vi "bazar.vi"() -> ()   [LabVIEW 2014]
uses:
  <userlib>/AndorSDK3/Data/GetPixelData16.vi
panel:
  out "Photoluminescence versus time":cluster{"X":dbl, "Y":dbl}[](graph)
  in  "Apply Settings":bool
  in  "Centre AOI":bool
  in  "AOI Width":i64
  in  "AOI Height":i64
  in  "Run":bool
  out "Ready":bool
  out "Intensity Graph":u16[][](graph)
  in  "error":errorcluster
  out "AOIStride":i64
  out "Pixel Encoding":string
  in  "PreAmp Gain Control":string(combo)
  out "PixelData":u16[](array[numeric])
  out "ByteData":u8[](array[numeric])
  in  "ExposureTime":dbl=0.1
  out "ImageSizeBytes":i64
  out "Handle":i32
  in  "Set CW Light":bool
  in  "Technical parameters":enum32{"Aardvark", "762 Address", "Errors"}(tab)
  out "Bit Rate":i16
  out "Aardvark Power Enable":bool
  out "Pullup?":bool
  in  "Num Bytes to Fetch (64)":u8=64 min=1
  in  "Address (0x50)":u16=80 max=1023 format="%.0x"
  in  "error in (no error)":errorcluster
  out "error out":errorcluster
  in  "Disabel Output":bool
  out "Light ON":bool
  in  "Enable Ouput":bool
  in  "Dark Time":dbl
  in  "Pulse Period":dbl
  in  "Pulse Width":dbl
  in  "Laser Current (A)":dbl
  in  "Set Config.":bool
  in  "Read Current Config.":bool
  out "Dark Time":dbl
  out "Pulse Period":dbl
  out "Pulse Width":dbl
  out "Laser Current (A)":dbl
  # "Pulsed Light"
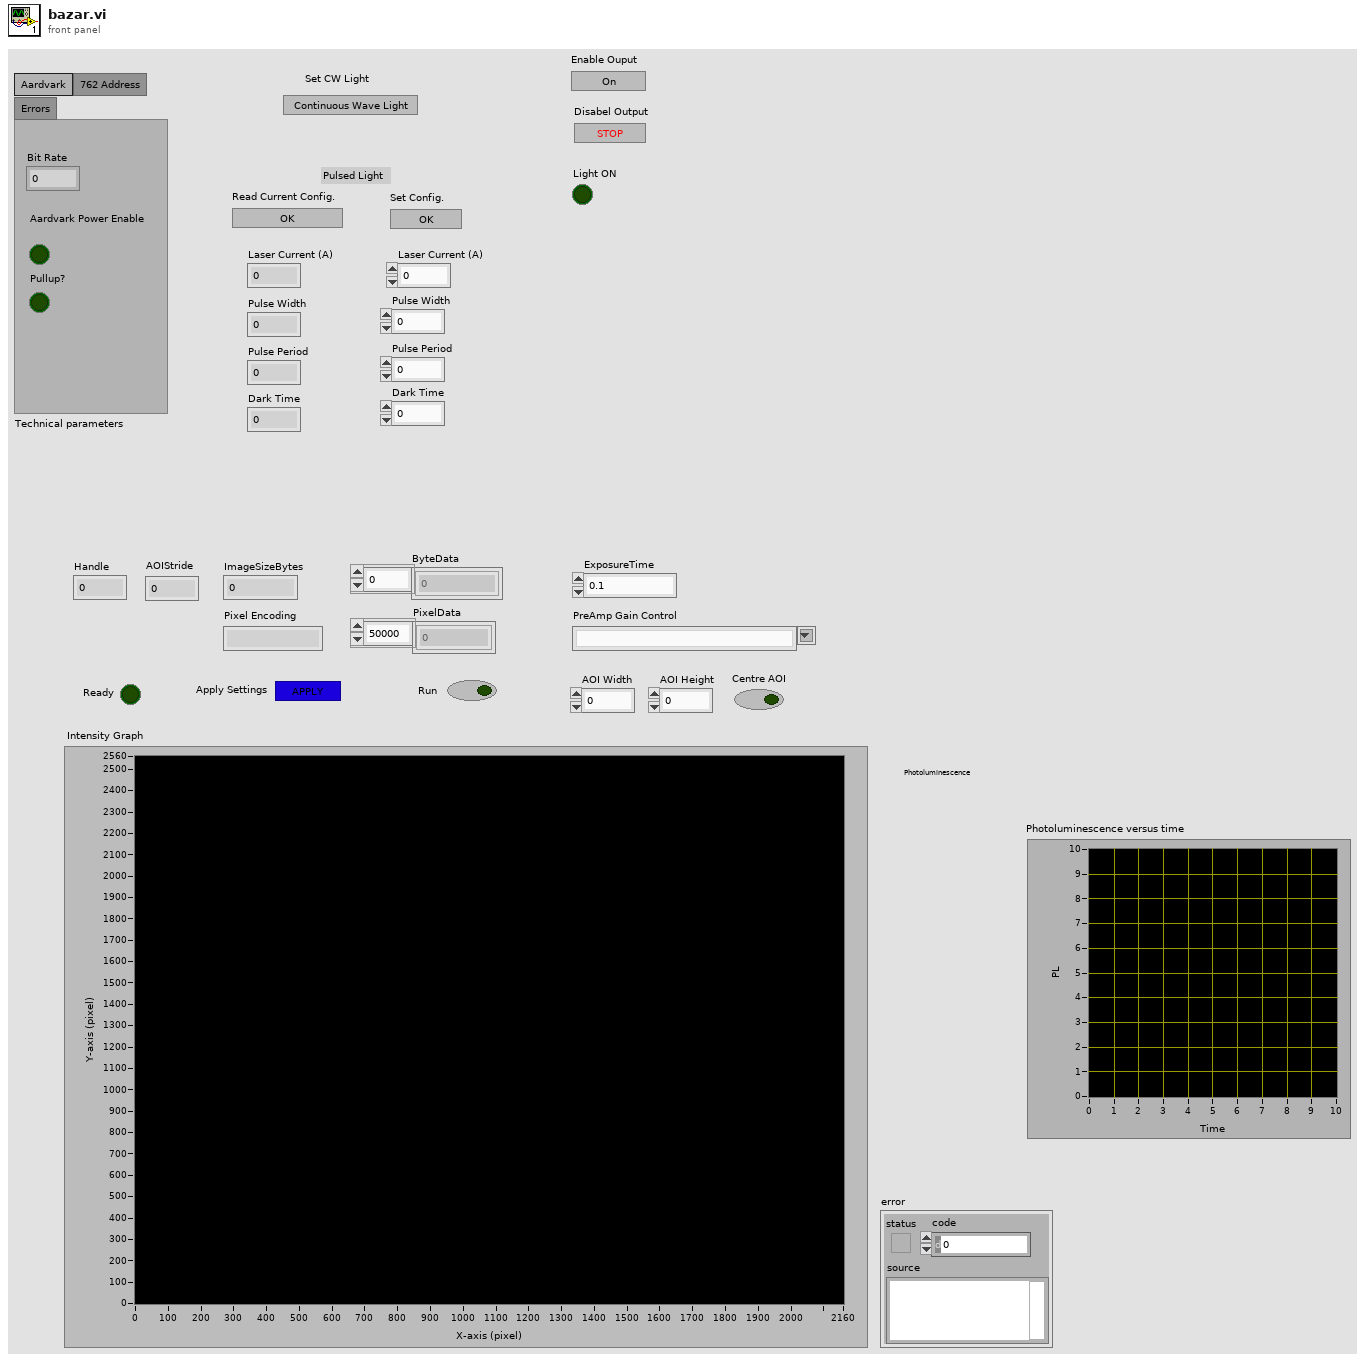
[diagram p1: front panel]
types:
  T1 = enum8{"Enabled", "Disabled", "Disabled and Grayed Out"}
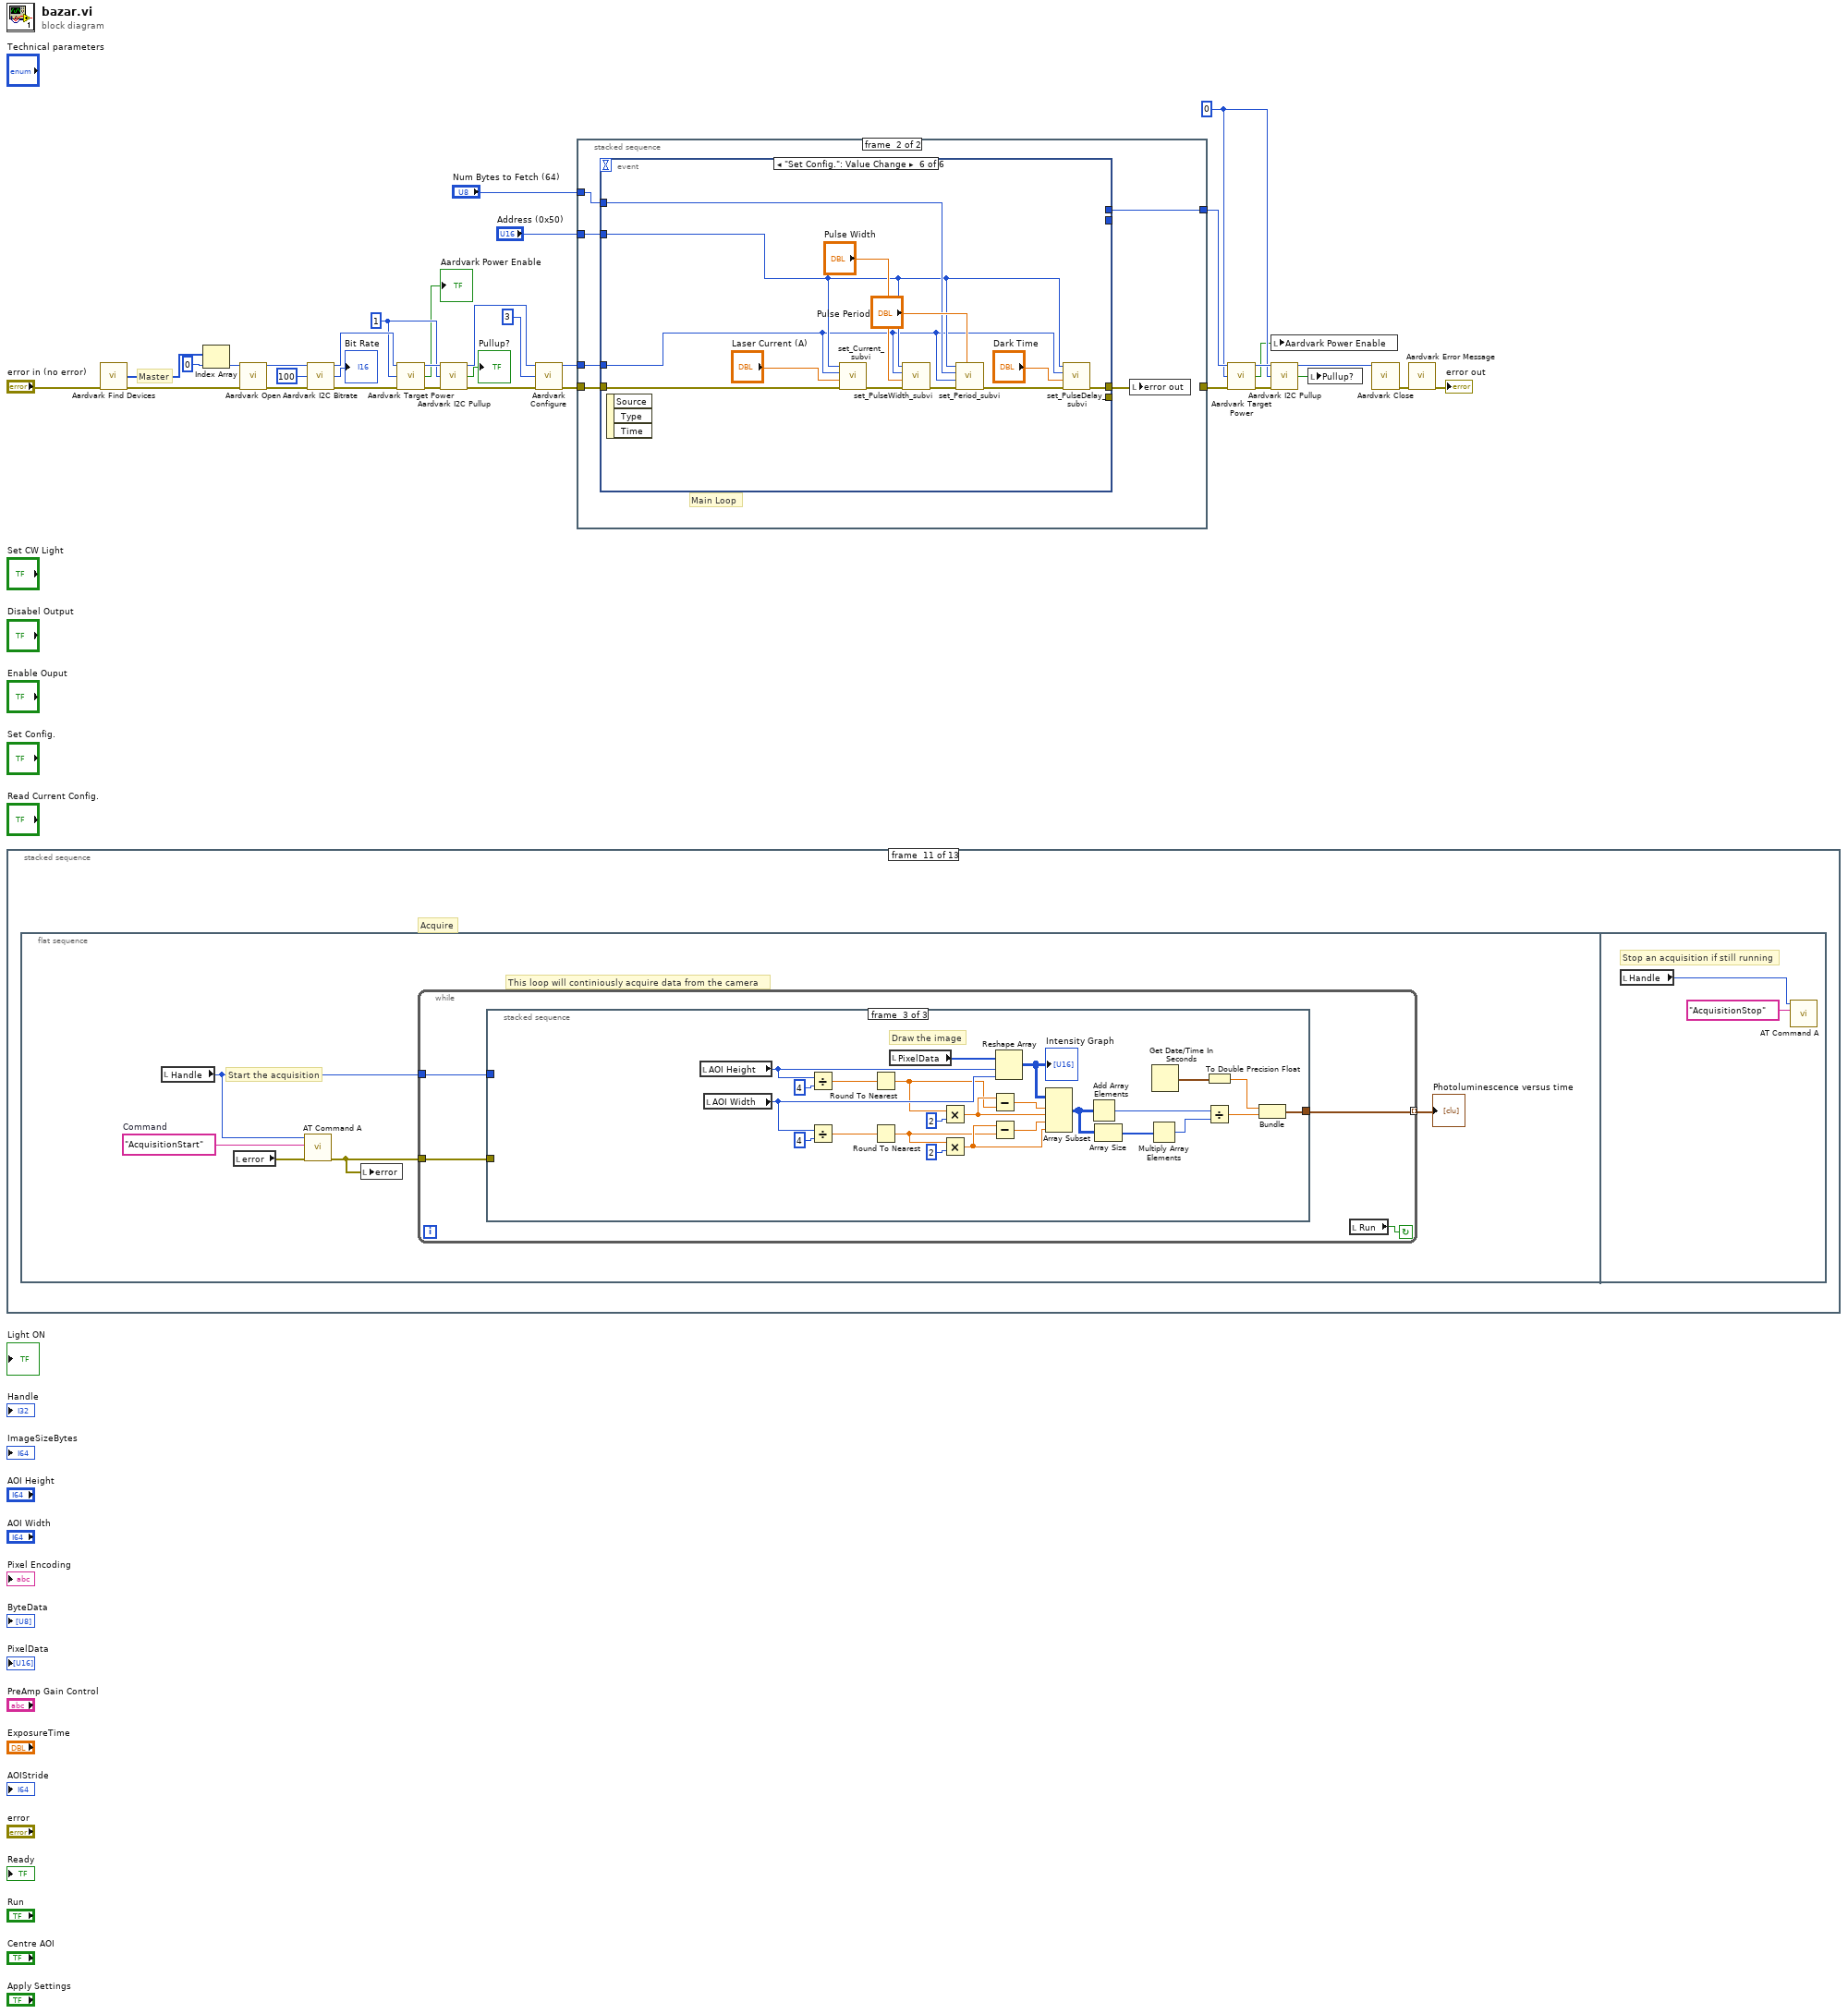
[diagram p0: block diagram]
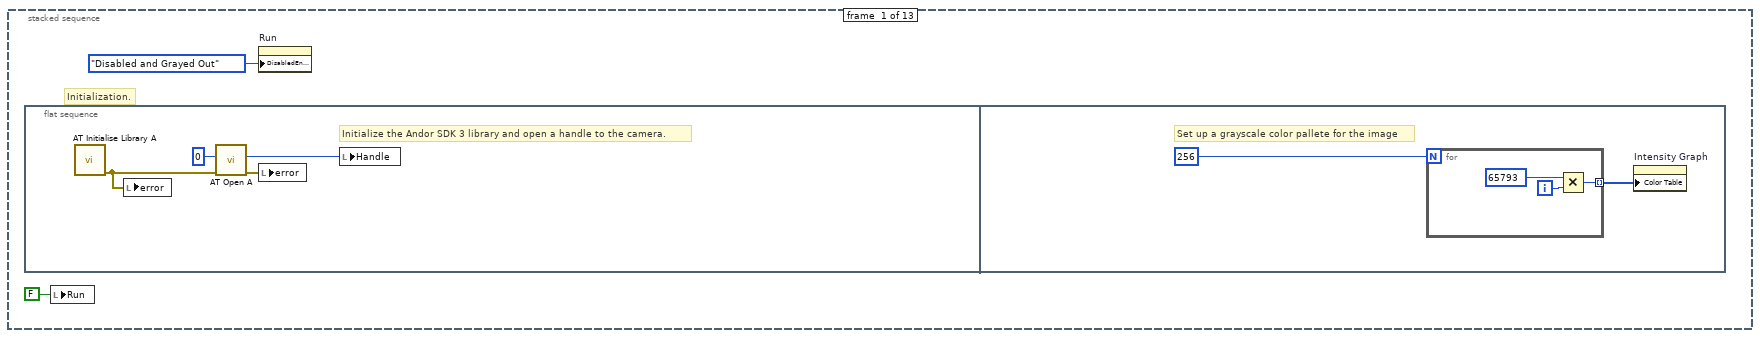
[diagram p2: hidden frame]
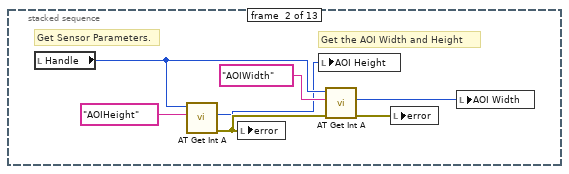
[diagram p3: hidden frame]
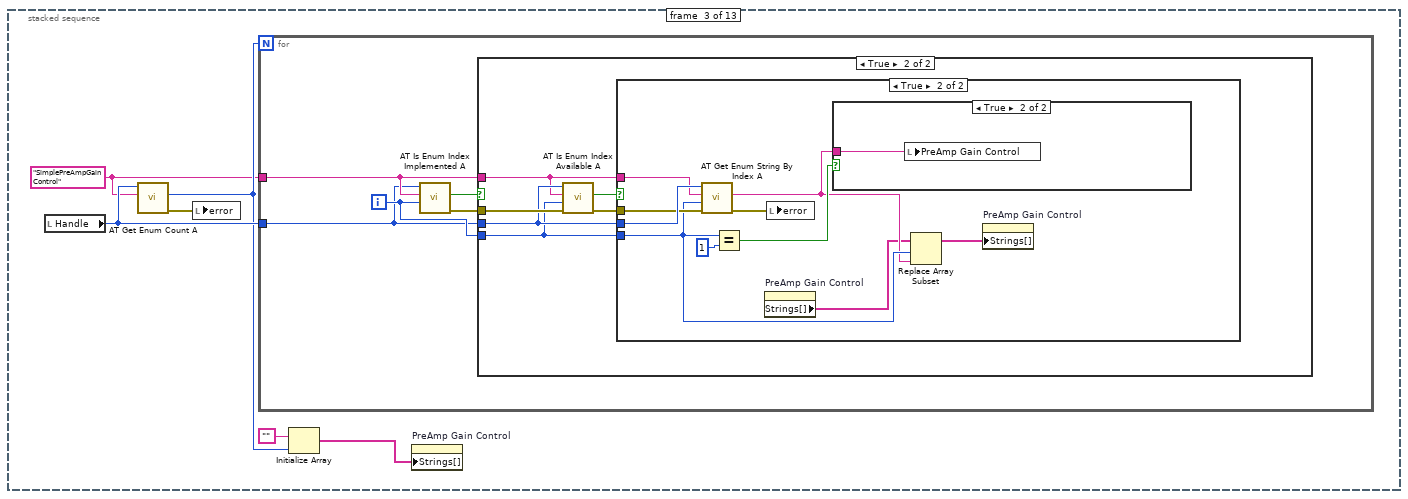
[diagram p4: hidden frame]
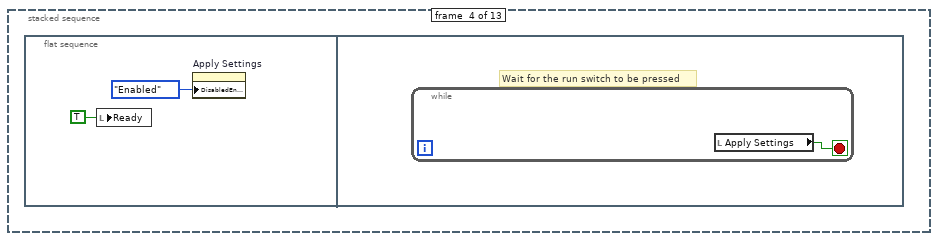
[diagram p8: hidden frame]
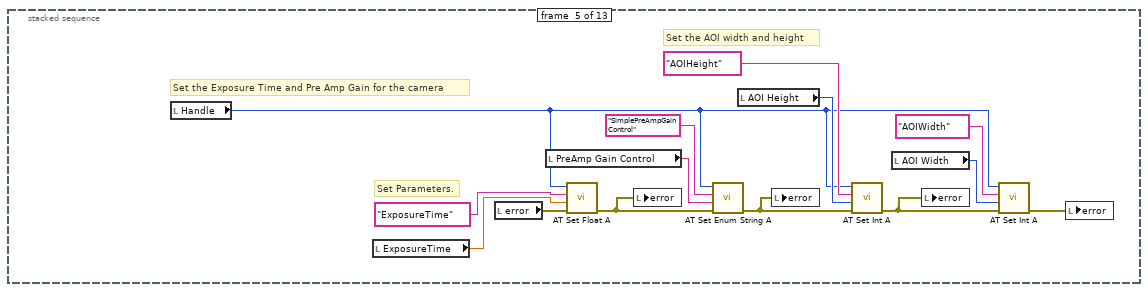
[diagram p9: hidden frame]
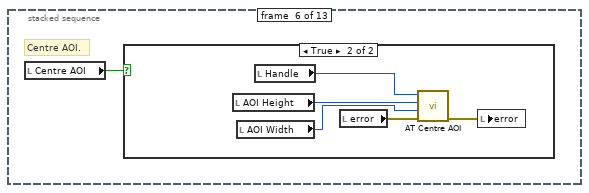
[diagram p10: hidden frame]
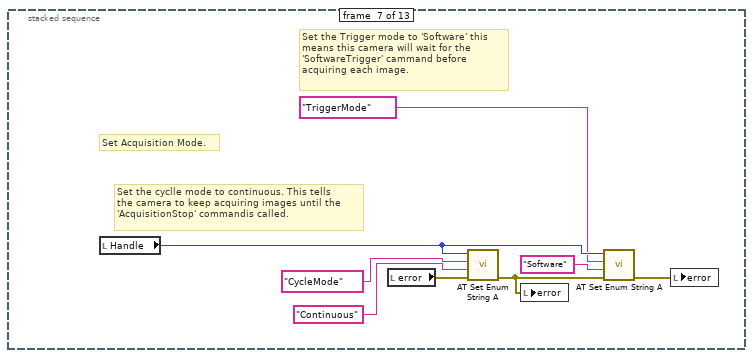
[diagram p12: hidden frame]
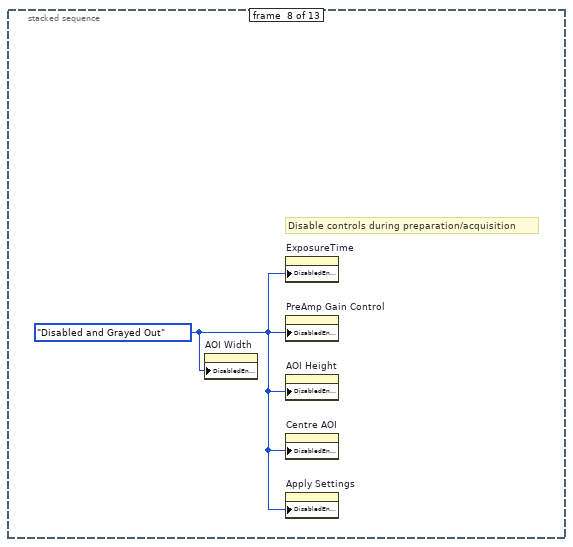
[diagram p13: hidden frame]
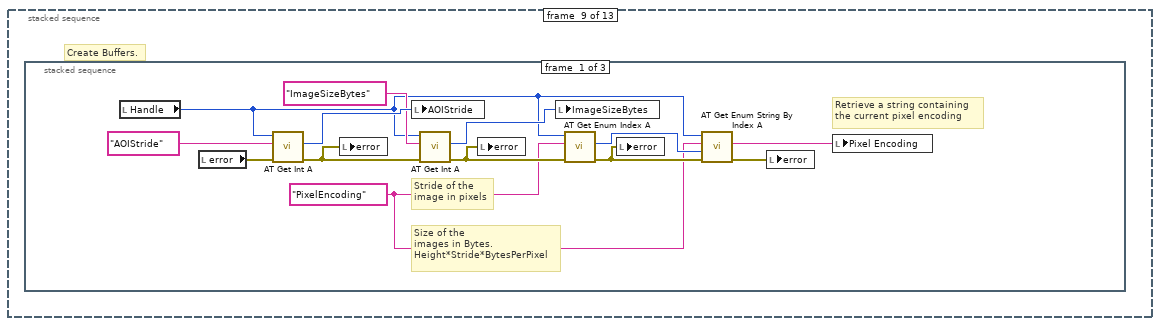
[diagram p14: hidden frame]
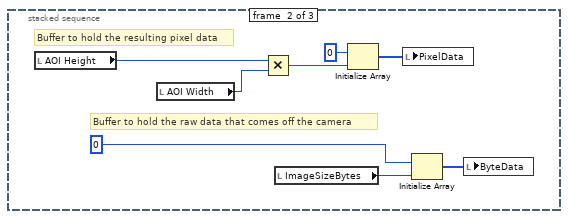
[diagram p15: hidden frame]
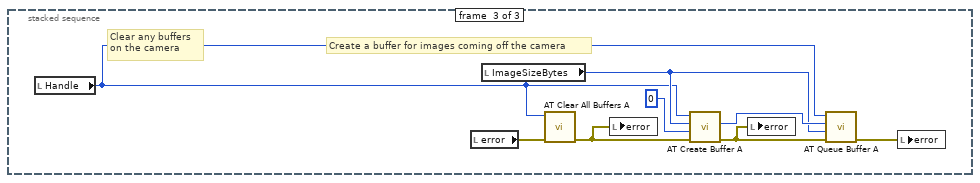
[diagram p16: hidden frame]
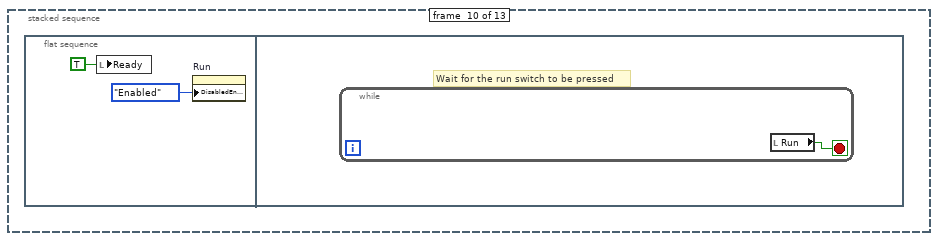
[diagram p17: hidden frame]
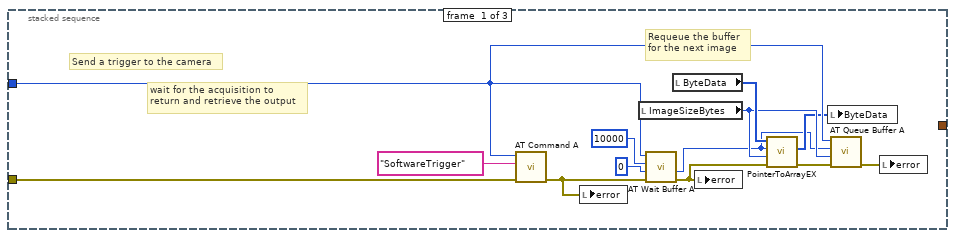
[diagram p18: hidden frame]
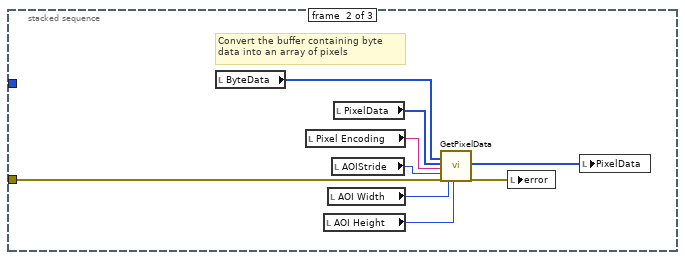
[diagram p19: hidden frame]
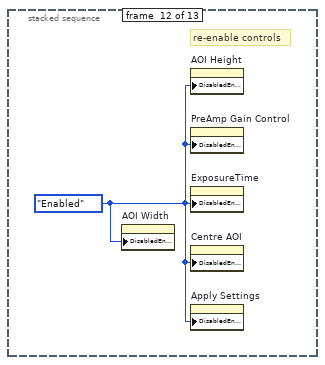
[diagram p20: hidden frame]
diagram:
  w3 = 0
  w13 = 1
  # "Master"
  n1 = stacked-sequence {
    frame #0 {
      # "Initialization."
      n2 = flat-sequence {
        frame #0 {
          # "Initialize the Andor SDK 3 library and open a handle to the camera."
          n3 = call <userlib>:"AT Initialise Library A.vi"() -> ("error out"=w37:errorcluster)  [unwired: 10 in, 1 out]
          n4 = local write "error"(w37) -> ()
          n5 = call <userlib>:"AT Open A.vi"("error in (no error)"=w37, "CameraIndex"=0) -> ("error out"=w36:errorcluster, "Handle"=w38:i32)  [unwired: 7 in, 1 out]
          n6 = local write "error"(w36) -> ()
          n7 = local write "Handle"(w38) -> ()
        }
        frame #1 {
          # "Set up a grayscale color pallete for the image"
          n8 = for {
            N: 256 -> [_]
            tunnel: [w43] -> w40 mode=indexing
            i -> [w44]
            n9 = Multiply(x=65793, y=w44) -> (x*y=w43:i32)
          }
          n10 = property on="Intensity Graph" class="IntGraph (strict)"("Color Table"=w40) -> ()  [unwired: 2 in, 2 out]
        }
      }
      n11 = local write "Run"(FALSE ("Run")) -> ()
      n12 = property on="Run" class="Bool (strict)"("DisabledEnum"=T1."Disabled and Grayed Out" ("Disabled")) -> ()  [unwired: 2 in, 2 out]
    }
    frame #1 {
      # "Get the AOI Width and Height"
      # "Get Sensor Parameters."
      n13 = local read "Handle"() -> (w48:i32)
      n14 = call <userlib>:"AT Get Int A.vi"("Feature"="AOIHeight" ("Integer feature 2"), "Handle"=w48) -> ("error out"=w47:errorcluster, "Value"=w45:i64)  [unwired: 7 in, 1 out]
      n15 = local write "error"(w47) -> ()
      n16 = local write "AOI Height"(w45) -> ()
      n17 = call <userlib>:"AT Get Int A.vi"("error in (no error)"=w47, "Feature"="AOIWidth" ("Integer feature"), "Handle"=w48) -> ("error out"=w51:errorcluster, "Value"=w46:i64)  [unwired: 6 in, 1 out]
      n18 = local write "error"(w51) -> ()
      n19 = local write "AOI Width"(w46) -> ()
    }
    frame #2 {
      w52 = "SimplePreAmpGainControl" ("Enum feature")
      n20 = local read "Handle"() -> (w56:i32)
      n21 = call <userlib>:"AT Get Enum Count A.vi"("Feature"=w52, "Handle"=w56) -> ("error out"=w57:errorcluster, "Count"=w55:i32)  [unwired: 7 in, 1 out]
      n22 = local write "error"(w57) -> ()
      n23 = for {
        N: w55 -> [_]
        tunnel: w56 -> [w59]
        tunnel: w52 -> [w60]
        i -> [w61]
        n24 = call <userlib>:"AT Is Enum Index Implemented A.vi"("Index"=w61, "Feature"=w60, "Handle"=w59) -> ("error out"=w58:errorcluster, "Implemented"=w62:bool)  [unwired: 6 in, 1 out]
        n25 = case shown="True" w62 {
          tunnel: w61 -> [_ w64]
          tunnel: w60 -> [_ w65]
          tunnel: w59 -> [_ w66]
          tunnel: w58 -> [_ w68]
          frame False {
          }
          frame True {
            n26 = call <userlib>:"AT Is Enum Index Available A.vi"("error in (no error)"=w68, "Index"=w64, "Feature"=w65, "Handle"=w66) -> ("error out"=w63:errorcluster, "Available"=w67:bool)  [unwired: 5 in, 1 out]
            n27 = case shown="True" w67 {
              tunnel: w66 -> [_ w78]
              tunnel: w65 -> [_ w77]
              tunnel: w64 -> [_ w74]
              tunnel: w63 -> [_ w76]
              frame False {
              }
              frame True {
                n28 = call <userlib>:"AT Get Enum String By Index A.vi"("error in (no error)"=w76, "Index"=w74, "Feature"=w77, "Handle"=w78) -> ("error out"=w75:errorcluster, "String"=w71:string)  [unwired: 5 in, 1 out]
                n29 = Equal?(x=w74, y=1) -> (x = y?=w72:bool)
                n30 = property on="PreAmp Gain Control" class="CmbBox"() -> ("Strings[]"=w70:string[])  [unwired: 2 in, 2 out]
                n31 = local write "error"(w75) -> ()
                n32 = case shown="True" w72 {
                  tunnel: w71 -> [_ w79]
                  frame False {
                  }
                  frame True {
                    n33 = local write "PreAmp Gain Control"(w79) -> ()
                  }
                }
                n34 = Replace Array Subset(array=w70, new element=w71, index=w74) -> (w69:string[])
                n35 = property on="PreAmp Gain Control" class="CmbBox"("Strings[]"=w69) -> ()  [unwired: 2 in, 2 out]
              }
            }
          }
        }
      }
      n36 = Initialize Array("", w55) -> (w53:string[])
      n37 = property on="PreAmp Gain Control" class="CmbBox"("Strings[]"=w53) -> ()  [unwired: 2 in, 2 out]
    }
    frame #3 {
      n38 = flat-sequence {
        frame #0 {
          n39 = local write "Ready"(TRUE ("Ready")) -> ()
          n40 = property on="Apply Settings" class="Bool (strict)"("DisabledEnum"=T1."Enabled" ("Disabled")) -> ()  [unwired: 2 in, 2 out]
        }
        frame #1 {
          # "Wait for the run switch to be pressed"
          n41 = while {
            stop <- w82 stop-if-true
            n42 = local read "Apply Settings"() -> (w82:bool)
          }
        }
      }
    }
    frame #4 {
      # "Set the AOI width and height"
      # "Set the Exposure Time and Pre Amp Gain for the camera"
      # "Set Parameters."
      n43 = local read "Handle"() -> (w84:i32)
      n44 = local read "ExposureTime"() -> (w96:dbl)
      n45 = local read "error"() -> (w92:errorcluster)
      n46 = local read "PreAmp Gain Control"() -> (w95:string)
      n47 = call <userlib>:"AT Set Float A.vi"("error in (no error)"=w92, "Value"=w96, "Feature"="ExposureTime" ("ExposureTime"), "Hndl"=w84) -> ("error out"=w94:errorcluster)  [unwired: 6 in, 1 out]
      n48 = local write "error"(w94) -> ()
      n49 = call <userlib>:"AT Set Enum String A.vi"("error in (no error)"=w94, "String"=w95, "Feature"="SimplePreAmpGainControl" ("Enum feature"), "Handle"=w84) -> ("error out"=w91:errorcluster)  [unwired: 6 in, 1 out]
      n50 = local read "AOI Height"() -> (w88:i64)
      n51 = local write "error"(w91) -> ()
      n52 = call <userlib>:"AT Set Int A.vi"("error in (no error)"=w91, "Value"=w88, "Feature"="AOIHeight" ("Integer feature"), "Handle"=w84) -> ("error out"=w89:errorcluster)  [unwired: 6 in, 1 out]
      n53 = local read "AOI Width"() -> (w87:i64)
      n54 = local write "error"(w89) -> ()
      n55 = call <userlib>:"AT Set Int A.vi"("error in (no error)"=w89, "Value"=w87, "Feature"="AOIWidth" ("Integer feature 2"), "Handle"=w84) -> ("error out"=w90:errorcluster)  [unwired: 6 in, 1 out]
      n56 = local write "error"(w90) -> ()
    }
    frame #5 {
      # "Centre AOI."
      n57 = local read "Centre AOI"() -> (w97:bool)
      n58 = case shown="True" w97 {
        frame False {
        }
        frame True {
          n59 = local read "AOI Height"() -> (w99:i64)
          n60 = local read "AOI Width"() -> (w100:i64)
          n61 = local read "Handle"() -> (w98:i32)
          n62 = local read "error"() -> (w101:errorcluster)
          n63 = call <userlib>:"AT Centre AOI.vi"("error in (no error)"=w101, "AOI Width"=w100, "AOI Height"=w99, "Handle"=w98) -> ("error out"=w102:errorcluster)  [unwired: 7 in]
          n64 = local write "error"(w102) -> ()
        }
      }
    }
    frame #6 {
      # "Set the Trigger mode to 'Software' this \nmeans this camera will wait for the \n'SoftwareTrigger' cammand before \nacquiring each image."
      # "Set the cyclle mode to continuous. This tells \nthe camera to keep acquiring images until the \n'AcquisitionStop' commandis called."
      # "Set Acquisition Mode."
      n65 = local read "Handle"() -> (w107:i32)
      n66 = local read "error"() -> (w109:errorcluster)
      n67 = call <userlib>:"AT Set Enum String A.vi"("error in (no error)"=w109, "String"="Continuous", "Feature"="CycleMode" ("Enum feature"), "Handle"=w107) -> ("error out"=w108:errorcluster)  [unwired: 6 in, 1 out]
      n68 = local write "error"(w108) -> ()
      n69 = call <userlib>:"AT Set Enum String A.vi"("error in (no error)"=w108, "String"="Software", "Feature"="TriggerMode" ("Enum feature"), "Handle"=w107) -> ("error out"=w105:errorcluster)  [unwired: 6 in, 1 out]
      n70 = local write "error"(w105) -> ()
    }
    frame #7 {
      w111 = T1."Disabled and Grayed Out" ("Disabled")
      # "Disable controls during preparation/acquisition"
      n71 = property on="AOI Width" class="DigNum (strict)"("DisabledEnum"=w111) -> ()  [unwired: 2 in, 2 out]
      n72 = property on="ExposureTime" class="DigNum (strict)"("DisabledEnum"=w111) -> ()  [unwired: 2 in, 2 out]
      n73 = property on="PreAmp Gain Control" class="CmbBox"("DisabledEnum"=w111) -> ()  [unwired: 2 in, 2 out]
      n74 = property on="AOI Height" class="DigNum (strict)"("DisabledEnum"=w111) -> ()  [unwired: 2 in, 2 out]
      n75 = property on="Centre AOI" class="Bool (strict)"("DisabledEnum"=w111) -> ()  [unwired: 2 in, 2 out]
      n76 = property on="Apply Settings" class="Bool (strict)"("DisabledEnum"=w111) -> ()  [unwired: 2 in, 2 out]
    }
    frame #8 {
      # "Create Buffers."
      n77 = stacked-sequence {
        frame #0 {
          w112 = "PixelEncoding" ("Enum feature")
          # "Retrieve a string containing \nthe current pixel encoding"
          # "Stride of the\nimage in pixels"
          # "Size of the\nimages in Bytes.\nHeight*Stride*BytesPerPixel"
          n78 = local read "Handle"() -> (w114:i32)
          n79 = local read "error"() -> (w113:errorcluster)
          n80 = call <userlib>:"AT Get Int A.vi"("error in (no error)"=w113, "Feature"="AOIStride" ("Integer feature"), "Handle"=w114) -> ("error out"=w120:errorcluster, "Value"=w124:i64)  [unwired: 6 in, 1 out]
          n81 = local write "error"(w120) -> ()
          n82 = local write "AOIStride"(w124) -> ()
          n83 = call <userlib>:"AT Get Int A.vi"("error in (no error)"=w120, "Feature"="ImageSizeBytes" ("Integer feature"), "Handle"=w114) -> ("error out"=w119:errorcluster, "Value"=w123:i64)  [unwired: 6 in, 1 out]
          n84 = local write "error"(w119) -> ()
          n85 = local write "ImageSizeBytes"(w123) -> ()
          n86 = call <userlib>:"AT Get Enum Index A.vi"("error in (no error)"=w119, "Feature"=w112, "Handle"=w114) -> ("error out"=w118:errorcluster, "Value"=w117:i32)  [unwired: 6 in, 1 out]
          n87 = local write "error"(w118) -> ()
          n88 = call <userlib>:"AT Get Enum String By Index A.vi"("error in (no error)"=w118, "Index"=w117, "Feature"=w112, "Handle"=w114) -> ("error out"=w115:errorcluster, "String"=w116:string)  [unwired: 5 in, 1 out]
          n89 = local write "error"(w115) -> ()
          n90 = local write "Pixel Encoding"(w116) -> ()
        }
        frame #1 {
          # "Buffer to hold the resulting pixel data"
          # "Buffer to hold the raw data that comes off the camera"
          n91 = local read "AOI Height"() -> (w130:i64)
          n92 = local read "AOI Width"() -> (w131:i64)
          n93 = Multiply(x=w130, y=w131) -> (x*y=w125:i64)
          n94 = local read "ImageSizeBytes"() -> (w126:i64)
          n95 = Initialize Array(i64 0, w125) -> (w129:i64[])
          n96 = local write "PixelData"(w129) -> ()
          n97 = Initialize Array(u8 0, w126) -> (w128:u8[])
          n98 = local write "ByteData"(w128) -> ()
        }
        frame #2 {
          # "Clear any buffers \non the camera"
          # "Create a buffer for images coming off the camera"
          n99 = local read "Handle"() -> (w133:i32)
          n100 = local read "error"() -> (w135:errorcluster)
          n101 = local read "ImageSizeBytes"() -> (w137:i64)
          n102 = call <userlib>:"AT Clear All Buffers A.vi"("error in (no error)"=w135, "Handle"=w133) -> ("error out"=w134:errorcluster)  [unwired: 8 in, 1 out]
          n103 = local write "error"(w134) -> ()
          n104 = call <userlib>:"AT Create Buffer A.vi"("error in (no error)"=w134, "Buffer"=0 ("Size"), "Size"=w137, "Handle"=w133) -> ("error out"=w139:errorcluster, "Buffer out"=w140:u64)  [unwired: 5 in, 1 out]
          n105 = local write "error"(w139) -> ()
          n106 = call <userlib>:"AT Queue Buffer A.vi"("error in (no error)"=w139, "PtrSize"=w137, "Ptr"=w140, "Handle"=w133) -> ("error out"=w136:errorcluster)  [unwired: 6 in, 1 out]
          n107 = local write "error"(w136) -> ()
        }
      }
    }
    frame #9 {
      n108 = flat-sequence {
        frame #0 {
          n109 = local write "Ready"(TRUE ("Ready")) -> ()
          n110 = property on="Run" class="Bool (strict)"("DisabledEnum"=T1."Enabled" ("Disabled")) -> ()  [unwired: 2 in, 2 out]
        }
        frame #1 {
          # "Wait for the run switch to be pressed"
          n111 = while {
            stop <- w143 stop-if-true
            n112 = local read "Run"() -> (w143:bool)
          }
        }
      }
    }
    frame #10 {
      # "Acquire"
      n113 = flat-sequence {
        frame #0 {
          w146 = "AcquisitionStart"  # Command
          # "This loop will continiously acquire data from the camera"
          # "Start the acquisition"
          n114 = local read "Handle"() -> (w148:i32)
          n115 = local read "error"() -> (w147:errorcluster)
          n116 = call <userlib>:"AT Command A.vi"("error in (no error)"=w147, "Feature"=w146, "Handle"=w148) -> ("error out"=w145:errorcluster)  [unwired: 7 in, 1 out]
          n117 = local write "error"(w145) -> ()
          n118 = while {
            tunnel: w148 -> [w151]
            tunnel: w145 -> [w152]
            tunnel: [w149] -> w144 mode=indexing
            stop <- w150 continue-if-true
            n119 = stacked-sequence {
              tunnel: w152 -> [w160 w166 _]
              tunnel: w151 -> [w161 _ _]
              tunnel: [_ _ w175] -> w149
              frame #0 {
                # "Requeue the buffer\nfor the next image"
                # "Send a trigger to the camera"
                # "wait for the acquisition to \nreturn and retrieve the output"
                n120 = call <userlib>:"AT Command A.vi"("error in (no error)"=w160, "Feature"="SoftwareTrigger" ("Command"), "Handle"=w161) -> ("error out"=w159:errorcluster)  [unwired: 7 in, 1 out]
                n121 = local write "error"(w159) -> ()
                n122 = local read "ImageSizeBytes"() -> (w157:i64)
                n123 = call <userlib>:"AT Wait Buffer A.vi"("error in (no error)"=w159, "Input buffer"=u32 0, "Timeout"=u32 10000, "Handle"=w161) -> ("error out"=w154:errorcluster, "Output buffer"=w153:u64)  [unwired: 4 in, 2 out]
                n124 = local read "ByteData"() -> (w158:u8[])
                n125 = local write "error"(w154) -> ()
                n126 = call <userlib>:"PointerToArrayEX.vi"("Array in"=w158, "Pointer In"=w153, "Pointer Size"=w157, "error in (no error)"=w154) -> ("Array out"=w156:u8[], "error out"=w155:errorcluster)  [unwired: 4 in]
                n127 = local write "ByteData"(w156) -> ()
                n128 = call <userlib>:"AT Queue Buffer A.vi"("error in (no error)"=w155, "PtrSize"=w157, "Ptr"=w153, "Handle"=w161) -> ("error out"=w163:errorcluster)  [unwired: 6 in, 1 out]
                n129 = local write "error"(w163) -> ()
              }
              frame #1 {
                # "Convert the buffer containing byte \ndata into an array of pixels"
                n130 = local read "ByteData"() -> (w167:u8[])
                n131 = local read "Pixel Encoding"() -> (w172:string)
                n132 = local read "AOI Height"() -> (w169:i64)
                n133 = local read "AOI Width"() -> (w170:i64)
                n134 = local read "AOIStride"() -> (w173:i64)
                n135 = local read "PixelData"() -> (w171:u16[])
                n136 = call-poly <userlib>:"GetPixelData.vi"("Input buffer"=w167, "Output buffer in"=w171, "Pixel Encoding"=w172, "Stride"=w173, "error in (no error)"=w166, "Width"=w170, "Height"=w169) -> ("Output buffer out"=w174:u16[], "error out"=w168:errorcluster)  [unwired: 10 in, 1 out]
                n137 = local write "error"(w168) -> ()
                n138 = local write "PixelData"(w174) -> ()
              }
              frame #2 {
                # "Draw the image"
                n139 = local read "AOI Height"() -> (w196:i64)
                n140 = local read "AOI Width"() -> (w189:i64)
                n141 = Divide(x=w196, y=4) -> (x/y=w182:dbl)
                n142 = Divide(x=w189, y=4) -> (x/y=w180:dbl)
                n143 = Round To Nearest(number=w182) -> (nearest integer value=w181:dbl)
                n144 = Round To Nearest(number=w180) -> (nearest integer value=w179:dbl)
                n145 = local read "PixelData"() -> (w198:u16[])
                n146 = Multiply(x=w181, y=2) -> (x*y=w192:dbl)
                n147 = Multiply(x=w179, y=2) -> (x*y=w187:dbl)
                n148 = Subtract(x=w192, y=w181) -> (x-y=w193:dbl)
                n149 = Subtract(x=w187, y=w179) -> (x-y=w188:dbl)
                n150 = Reshape Array(w198, w196, w189) -> (w197:u16[][])
                "Intensity Graph" <- w197
                n151 = Array Subset(array=w197, index (row)=w193, length (row)=w192, index (col)=w188, length (col)=w187) -> (w186:u16[][])
                n152 = Add Array Elements(numeric array=w186) -> (sum=w184:u16)
                n153 = Array Size(array=w186) -> (size(s)=w185:i32[])
                n154 = Multiply Array Elements(1:w185) -> (0:w183:i32)
                n155 = Get Date/Time In Seconds() -> (seconds since 1Jan1904=w177:timestamp)
                n156 = To Double Precision Float(number=w177) -> (double precision float=w176:dbl)
                n157 = Divide(x=w184, y=w183) -> (x/y=w178:dbl)
                n158 = Bundle(w176, w178) -> (w175:cluster{dbl, dbl})  [unwired: 1 in]
              }
            }
            n159 = local read "Run"() -> (w150:bool)
          }
          "Photoluminescence versus time" <- w144
        }
        frame #1 {
          # "Stop an acquisition if still running"
          n160 = local read "Handle"() -> (w200:i32)
          n161 = call <userlib>:"AT Command A.vi"("Feature"="AcquisitionStop" ("Command"), "Handle"=w200) -> ()  [unwired: 8 in, 2 out]
        }
      }
    }
    frame #11 {
      w201 = T1."Enabled" ("Disabled")
      # "re-enable controls"
      n162 = property on="AOI Width" class="DigNum (strict)"("DisabledEnum"=w201) -> ()  [unwired: 2 in, 2 out]
      n163 = property on="AOI Height" class="DigNum (strict)"("DisabledEnum"=w201) -> ()  [unwired: 2 in, 2 out]
      n164 = property on="PreAmp Gain Control" class="CmbBox"("DisabledEnum"=w201) -> ()  [unwired: 2 in, 2 out]
      n165 = property on="ExposureTime" class="DigNum (strict)"("DisabledEnum"=w201) -> ()  [unwired: 2 in, 2 out]
      n166 = property on="Centre AOI" class="Bool (strict)"("DisabledEnum"=w201) -> ()  [unwired: 2 in, 2 out]
      n167 = property on="Apply Settings" class="Bool (strict)"("DisabledEnum"=w201) -> ()  [unwired: 2 in, 2 out]
    }
    frame #12 {
      # "Close the current camera handle and unload the library"
      # "ShutDown."
      n168 = local read "Handle"() -> (w204:i32)
      n169 = local write "Apply Settings"(FALSE ("Apply Settings")) -> ()
      n170 = local write "Ready"(FALSE ("Ready")) -> ()
      n171 = local read "error"() -> (w206:errorcluster)
      n172 = call <userlib>:"AT Flush A.vi"("error in (no error)"=w206, "Handle"=w204) -> ("error out"=w207:errorcluster)  [unwired: 8 in, 1 out]
      n173 = local write "error"(w207) -> ()
      n174 = call <userlib>:"AT Close A.vi"("error in (no error)"=w207, "Handle"=w204) -> ("error out"=w208:errorcluster)  [unwired: 8 in, 1 out]
      n175 = local write "error"(w208) -> ()
      n176 = call <userlib>:"AT Finalise Library A.vi"("error in (no error)"=w208) -> ("error out"=w205:errorcluster)  [unwired: 9 in, 1 out]
      n177 = local write "error"(w205) -> ()
    }
  }
  n178 = call <instrlib>:"Aardvark Find Devices.vi"("error in (no error)"="error in (no error)") -> ("Ports"=w32:u16[], "error out"=w31:errorcluster)  [unwired: 12 in, 1 out]
  n179 = Index Array(array=w32, index=0) -> (element=w30:u16)
  n180 = call <instrlib>:"Aardvark Open.vi"("Port Number (0)"=w30, "error in (no error)"=w31) -> ("Aardvark Handle"=w24:i32, "error out"=w20:errorcluster)  [unwired: 12 in]
  n181 = call <instrlib>:"Aardvark I2C Bitrate.vi"("Aardvark Handle"=w24, "Requested Bitrate kHz (100)"=100, "error in (no error)"=w20) -> ("dup Aardvark Handle"=w23:i32, "Actual Bitrate kHz"=→"Bit Rate":i32, "error out"=w19:errorcluster)  [unwired: 10 in]
  n182 = call <instrlib>:"Aardvark Target Power.vi"("Aardvark Handle"=w23, "Requested Configuration (2: Query)"=w13, "error in (no error)"=w19) -> ("dup Aardvark Handle"=w22:i32, "Target Power Enabled?"=→"Aardvark Power Enable":bool, "error out"=w18:errorcluster)  [unwired: 10 in]
  n183 = call <instrlib>:"Aardvark I2C Pullup.vi"("Aardvark Handle"=w22, "Requested Configuration (query)"=w13, "error in (no error)"=w18) -> ("dup Aardvark Handle"=w21:i32, "Pullups Enabled?"=→"Pullup?":bool, "error out"=w17:errorcluster)  [unwired: 10 in]
  n184 = call <instrlib>:"Aardvark Configure.vi"("Aardvark Handle"=w21, "Requested Configuration (0x80: Query)"=3, "error in (no error)"=w17) -> ("dup Aardvark Handle"=w15:i32, "error out"=w16:errorcluster)  [unwired: 10 in, 1 out]
  n185 = stacked-sequence {
    tunnel: w15 -> [w212 w221]
    tunnel: w16 -> [w215 w216]
    tunnel: [_ w220] -> w8
    tunnel: "Address (0x50)" -> [w210 w217]
    tunnel: "Num Bytes to Fetch (64)" -> [w211 w218]
    tunnel: [w209 _] -> w5
    frame #0 {
      # "Initialization of 762"
      n186 = call "disable_TEC_subvi.vi"("error in (no error)"=w215, "Aardvark Handle"=w212, "Num Bytes to Fetch (64) in"=w211, "Address (0x50) in"=w210) -> ("error out"=w214:errorcluster)  [unwired: 6 in, 1 out]
      n187 = call "enable_Config_subvi.vi"("error in (no error)"=w214, "Aardvark Handle"=w212, "Num Bytes to Fetch (64) in"=w211, "Address (0x50) in"=w210) -> ("error out"=w213:errorcluster)  [unwired: 6 in, 1 out]
      n188 = call "initDriver_setTrigger_softwareControl_subvi.vi"("error in (no error)"=w213, "Aardvark Handle"=w212, "Num Bytes to Fetch (64) in"=w211, "Address (0x50) in"=w210) -> ("error out"=w209:errorcluster)  [unwired: 7 in]
      n189 = local write "error out"(w209) -> ()
    }
    frame #1 {
      # "Main Loop"
      n190 = event shown="[5] \"Set Config.\": Value Change" {
        selector: _ -> [_ _ _ _ _ _]
        dyn-events: _ -> [_ _ _ _ _ _]
        timeout: _ -> [_ _ _ _ _ _]
        tunnel: w221 -> [_ w225 w232 w236 w243 w254]
        tunnel: w216 -> [_ w226 w231 w239 w244 w262]
        tunnel: [_ _ _ _ w243 _] -> _
        tunnel: [_ _ _ _ w242 _] -> _
        tunnel: [_ _ _ _ w243 _] -> w220
        tunnel: [_ w227 w230 w238 w242 w252] -> w219
        tunnel: w217 -> [_ w224 w233 w235 w241 w255]
        tunnel: w218 -> [_ w223 w234 w237 w240 w257]
        event Timeout {
          n191 = event-data() -> ()  [unwired: 1 in, 3 out]
        }
        event "Enable Ouput": Value Change {
          n192 = event-data() -> ()  [unwired: 1 in, 6 out]
          n193 = call "enable_Output_subvi.vi"("error in (no error)"=w226, "Aardvark Handle"=w225, "Num Bytes to Fetch (64) in"=w223, "Address (0x50) in"=w224) -> ("error out"=w227:errorcluster, "Light On"=w222:bool)  [unwired: 6 in]
          n194 = local write "Light ON"(w222) -> ()
        }
        event "Disabel Output": Value Change {
          n195 = event-data() -> ()  [unwired: 1 in, 6 out]
          n196 = call "disable_Output_subvi.vi"("error in (no error)"=w231, "Address (0x50) in"=w233, "Aardvark Handle"=w232, "Num Bytes to Fetch (64) in"=w234) -> ("error out"=w230:errorcluster, "Data Written"=w229:bool)  [unwired: 6 in]
          n197 = Not(x=w229) -> (.not. x?=w228:bool)
          n198 = local write "Light ON"(w228) -> ()
        }
        event "Set CW Light": Value Change {
          n199 = event-data() -> ()  [unwired: 1 in, 6 out]
          n200 = call "set_CW_light_subvi.vi"("error in (no error)"=w239, "Num Bytes to Fetch (64) in"=w237, "Aardvark Handle"=w236, "Address (0x50) in"=w235) -> ("error out"=w238:errorcluster)  [unwired: 7 in]
        }
        event "Read Current Config.": Value Change {
          n201 = event-data() -> ()  [unwired: 1 in, 6 out]
          n202 = call "read_Current_subvi.vi"("error in (no error)"=w244, "Address (0x50) in"=w241, "Aardvark Handle"=w243) -> ("error out"=w246:errorcluster, "Current"=→"Laser Current (A)":dbl)  [unwired: 7 in]
          n203 = call "read_Period_subvi.vi"("error in (no error)"=w246, "Address (0x50) in"=w241, "Num Bytes to Fetch (64) in"=w240, "Aardvark Handle"=w243) -> ("error out"=w248:errorcluster, "Period"=→"Pulse Period":dbl)  [unwired: 6 in]
          n204 = call "read_PulseDelay_subvi.vi"("error in (no error)"=w248, "Address (0x50) in"=w241, "Num Bytes to Fetch (64) in"=w240, "Aardvark Handle"=w243) -> ("error out"=w250:errorcluster, "PulseDelay"=→"Dark Time":dbl)  [unwired: 6 in]
          n205 = call "read_PulseWidth_subvi.vi"("error in (no error)"=w250, "Address (0x50) in"=w241, "Num Bytes to Fetch (64) in"=w240, "Aardvark Handle"=w243) -> ("error out"=w242:errorcluster, "PulseWidth"=→"Pulse Width":dbl)  [unwired: 6 in]
        }
        event "Set Config.": Value Change {
          n206 = event-data() -> ()  [unwired: 1 in, 3 out]
          n207 = call "set_Current_subvi.vi"("error in (no error)"=w262, "Current"="Laser Current (A)", "Aardvark Handle"=w254, "Address (0x50) in"=w255) -> ("error out"=w261:errorcluster)  [unwired: 7 in]
          n208 = call "set_PulseWidth_subvi.vi"("error in (no error)"=w261, "Pulsewidth"="Pulse Width", "Aardvark Handle"=w254, "Address (0x50) in"=w255) -> ("error out"=w259:errorcluster)  [unwired: 7 in]
          n209 = call "set_Period_subvi.vi"("Period"="Pulse Period", "error in (no error)"=w259, "Aardvark Handle"=w254, "Num Bytes to Fetch (64) in"=w257, "Address (0x50) in"=w255) -> ("error out"=w256:errorcluster)  [unwired: 6 in]
          n210 = call "set_PulseDelay_subvi.vi"("error in (no error)"=w256, "Pulse Delay"="Dark Time", "Aardvark Handle"=w254, "Address (0x50) in"=w255) -> ("error out"=w252:errorcluster)  [unwired: 7 in]
        }
      }
      n211 = local write "error out"(w219) -> ()
    }
  }
  n212 = call <instrlib>:"Aardvark Target Power.vi"("Aardvark Handle"=w8, "Requested Configuration (2: Query)"=w3, "error in (no error)"=w5) -> ("dup Aardvark Handle"=w7:i32, "Target Power Enabled?"=w2:bool, "error out"=w4:errorcluster)  [unwired: 10 in]
  n213 = local write "Aardvark Power Enable"(w2) -> ()
  n214 = call <instrlib>:"Aardvark I2C Pullup.vi"("Aardvark Handle"=w7, "Requested Configuration (query)"=w3, "error in (no error)"=w4) -> ("dup Aardvark Handle"=w6:i32, "Pullups Enabled?"=w1:bool)  [unwired: 10 in, 1 out]
  n215 = local write "Pullup?"(w1) -> ()
  n216 = call <instrlib>:"Aardvark Close.vi"("Aardvark Handle"=w6) -> ("error out"=w27:errorcluster)  [unwired: 14 in]
  n217 = call <instrlib>:"Aardvark Error Message.vi"("error in (no error)"=w27) -> ("error out"=→"error out":errorcluster)  [unwired: 10 in, 4 out]
